vi "Get Quads Center Color.vi"(5 "Index Array":u32[](array[numeric]), 6 "Alpha":sgl, 8 "Color Index Array":i32[](array[numeric]), 10 "Color Ramp Cluster":T2={"Color Ramp Style"=enum."None", "Color Ramp Array"=[16711934, 393471, 57855, 4390754, 16449346, 16744722, 16711680], "Color Ramp Index"=[45, 91, 133, 175, 219, 255], "Interpolate?"=FALSE, "Logarithm?"=FALSE}) -> (1 "Color Binding Mode":T1(ring), 3 "Color Array Out":cluster{"R":sgl, "G":sgl, "B":sgl, "A":sgl}[](array[cluster]))   [LabVIEW 2017, in "3D Surface.lvclass"]
uses:
  <vilib>/Math Plots/3D Math Plots/3D Surface/3D Surface/3D Surface.lvclass
  <vilib>/Math Plots/3D Math Plots/3D Plot/3D Plot/Typedef/Color Ramp Cluster.ctl
  <vilib>/Math Plots/3D Math Plots/3D Plot/3D Plot/3D Plot.lvclass
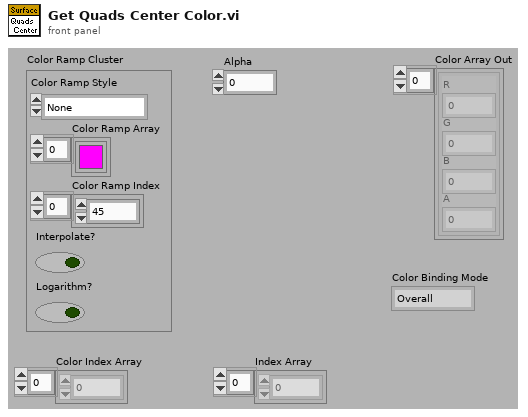
[diagram p1: front panel]
types:
  T1 = enum16{"Overall", "Per Primitive", "Per Vertex", "Binding Off"}
  T2 = typedef "3D Plot.lvclass/Color Ramp Cluster.ctl" = cluster{"Color Ramp Style":enum16{"None", "Shaded", "Color spectrum", "Grey scale", "Custom"}, "Color Ramp Array":u32[], "Color Ramp Index":i32[], "Interpolate?":bool, "Logarithm?":bool}
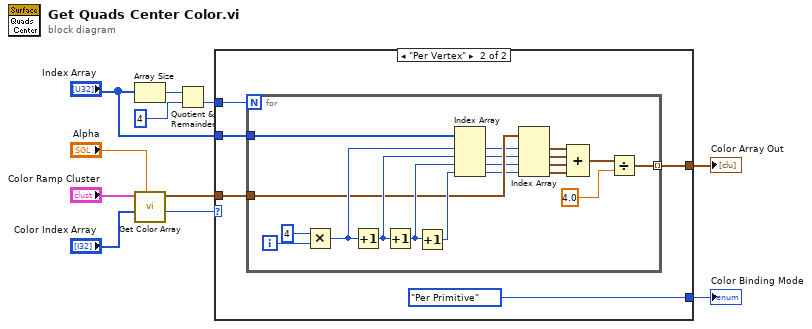
[diagram p0: block diagram]
diagram:
  n1 = Array Size(array="Index Array") -> (size(s)=w11:i32)
  n2 = call <vilib>:"Get Color Array.vi"("Alpha"="Alpha", "Color Index Array"="Color Index Array", "Color Ramp Cluster"="Color Ramp Cluster") -> ("Color Binding Mode"=w2:T1, "Color Array"=w6:cluster{"R":sgl, "G":sgl, "B":sgl, "A":sgl}[])  [unwired: 3 in, 4 out]
  n3 = Quotient & Remainder(x=w11, y=4) -> (floor(x/y)=w9:i32)  [unwired: 1 out]
  n4 = case shown="\"Per Vertex\"" w2 {
    selector: w2 -> [w12 _]
    tunnel: w9 -> [_ w18]
    tunnel: "Index Array" -> [_ w17]
    tunnel: w6 -> [w13 w16]
    tunnel: [w13 w15] -> w4
    tunnel: [w12 T1."Per Primitive" ("f")] -> w1
    frame Default {
    }
    frame "Per Vertex" {
      n5 = for {
        N: w18 -> [_]
        tunnel: w17 -> [w28]
        tunnel: [w29] -> w15 mode=indexing
        tunnel: w16 -> [w27]
        i -> [w36]
        n6 = Multiply(x=4 ("y"), y=w36) -> (x*y=w35:i32)
        n7 = Increment(x=w35) -> (x+1=w32:i32)
        n8 = Increment(x=w32) -> (x+1=w33:i32)
        n9 = Increment(x=w33) -> (x+1=w34:i32)
        n10 = Index Array(array=w28, index #1=w35, index #2=w32, index #3=w33, index #4=w34) -> (element #1=w26:u32, element #2=w25:u32, element #3=w24:u32, element #4=w23:u32)
        n11 = Index Array(array=w27, index #1=w26, index #2=w25, index #3=w24, index #4=w23) -> (element #1=w22:cluster{"R":sgl, "G":sgl, "B":sgl, "A":sgl}, element #2=w21:cluster{"R":sgl, "G":sgl, "B":sgl, "A":sgl}, element #3=w20:cluster{"R":sgl, "G":sgl, "B":sgl, "A":sgl}, element #4=w19:cluster{"R":sgl, "G":sgl, "B":sgl, "A":sgl})
        n12 = Compound Arithmetic op=ADD(w22, w21, w20, w19) -> (w31:cluster{"R":sgl, "G":sgl, "B":sgl, "A":sgl})
        n13 = Divide(x=w31, y=sgl 4.0) -> (x/y=w29:cluster{"R":sgl, "G":sgl, "B":sgl, "A":sgl})
      }
    }
  }
  "Color Binding Mode" <- w1
  "Color Array Out" <- w4
